vi "Post-Connect Action.vi"(8 "error in (no error)":errorcluster, 11 "Legacy Nested Endpoint in":refnum<class "Legacy Nested Endpoint.lvclass">) -> (0 "error out":errorcluster, 3 "Legacy Nested Endpoint out":refnum<class "Legacy Nested Endpoint.lvclass">)   [LabVIEW 2020, in "Legacy Nested Endpoint.lvlib" / "Legacy Nested Endpoint.lvclass"]
doc: "This overried sends a Connected message to this VI's caller."
uses:
  Legacy Nested Endpoint.lvclass
  <vilib>/ActorFramework/Actor/Actor.lvclass
  Legacy Nested Endpoint Messages/Connected Msg/Connected Msg.lvclass
  Nested Endpoint/Nested Endpoint/Nested Endpoint.lvclass
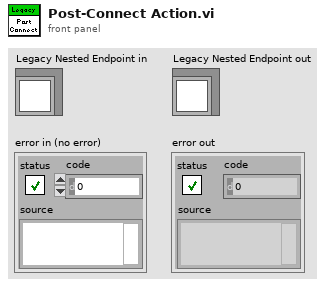
[diagram p1: front panel]
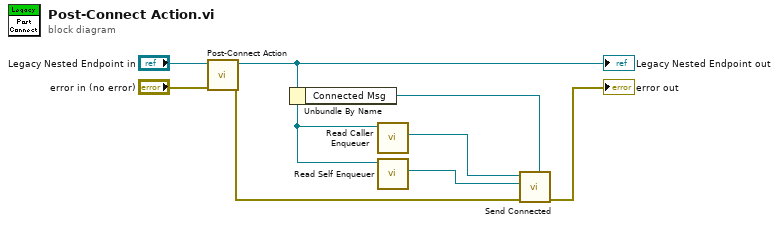
[diagram p0: block diagram]
diagram:
  n1 = call-parent "Post-Connect Action.vi"("error in (no error)"="error in (no error)", "Network Endpoint in"="Legacy Nested Endpoint in") -> ("error out"=w8:errorcluster, "Network Endpoint out"=w1:refnum<class "Legacy Nested Endpoint.lvclass">)  [unwired: 8 in]
  "Legacy Nested Endpoint out" <- w1
  n2 = Unbundle By Name(w1) -> ("Connected Msg"=w2:refnum<class "Connected Msg.lvclass">)
  n3 = call <vilib>:"Read Caller Enqueuer.vi"("Actor"=w1) -> ("Caller Enqueuer"=w4:refnum<class "Message Enqueuer.lvclass">)  [unwired: 10 in]
  n4 = call <vilib>:"Read Self Enqueuer.vi"("Actor"=w1) -> ("Self Enqueuer"=w3:refnum<class "Message Enqueuer.lvclass">)  [unwired: 10 in]
  n5 = call "Send Connected.vi"("Message Type"=w2, "error in (no error)"=w8, "Endpoint Enqueuer"=w3, "Message Enqueuer"=w4) -> ("error out"=→"error out":errorcluster)  [unwired: 6 in, 1 out]
